vi "Get Control Information.vi"(8 "error in (no error)":errorcluster, 11 "Boolean in":refnum<class "Boolean.lvclass">) -> (0 "error out":errorcluster, 2 "Control Information":string[][](array[string]), 3 "Boolean out":refnum<class "Boolean.lvclass">)   [LabVIEW 2017, in "Localization.lvlib" / "Boolean.lvclass"]
doc: "VI for override that is supposed to do go throgh the process for each control type and pull out the information that is necessary for each control.\n\nChoose Movement Consulting, LLC"
uses:
  Boolean.lvclass
  C:/Apps/CMC/OpenSource/Localization/Control Info/Control Info.lvclass
  Localization.lvlib
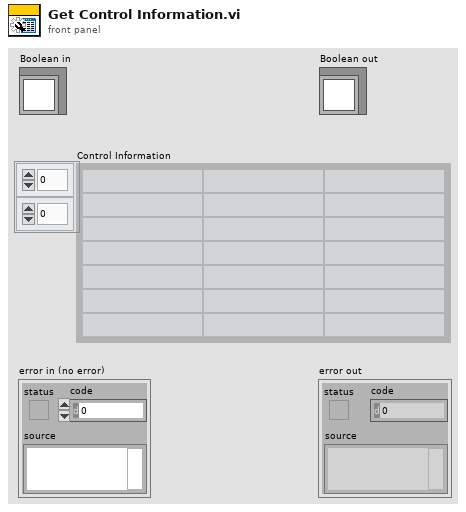
[diagram p1: front panel]
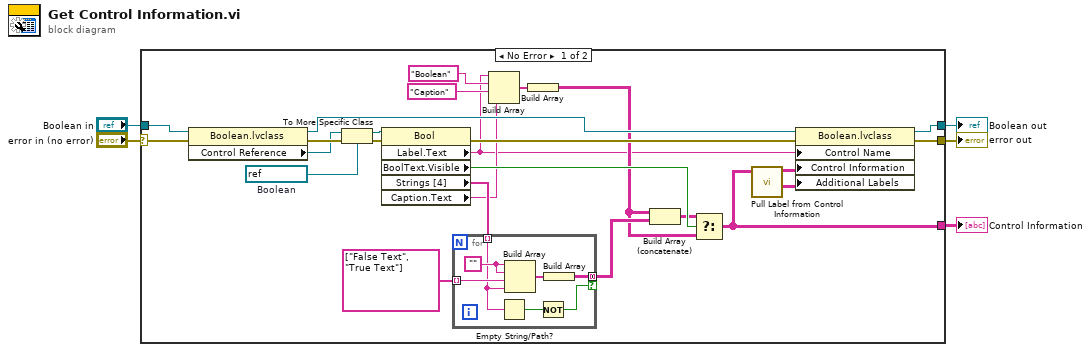
[diagram p0: block diagram]
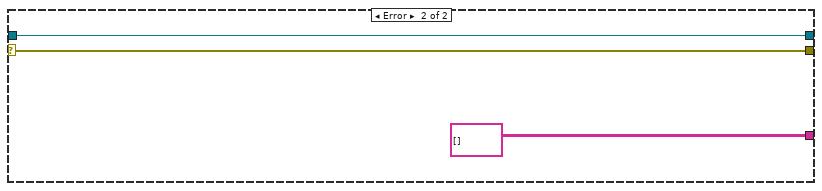
[diagram p2: hidden frame]
diagram:
  n1 = case shown="No Error" "error in (no error)" {
    selector: "error in (no error)" -> [w25 w40]
    tunnel: [w21 w40] -> w1
    tunnel: "Boolean in" -> [w24 w39]
    tunnel: [w9 string[][] []] -> w2
    tunnel: [w19 w39] -> w3
    frame No Error {
      w30 = refnum<vi> refnum  # Boolean
      n2 = property class="Boolean.lvclass"(reference=w24, error in=w25) -> (reference out=w20:refnum<class "Boolean.lvclass">, error out=w26:errorcluster, "Control Reference"=w23:refnum<vi>)
      n3 = To More Specific Class(target class=w30, reference=w23, error in=w26) -> (specific class reference=w29:refnum<vi>, error out=w27:errorcluster)
      n4 = property class="Bool"(reference=w29, error in=w27) -> (error out=w22:errorcluster, "Label.Text"=w6:string, "BoolText.Visible"=w18:bool, "Strings [4]"=w17:string[], "Caption.Text"=w10:string)  [unwired: 1 out]
      n5 = for {
        tunnel: w17 -> [w31] mode=indexing
        tunnel: string[] ["False Text", "True Text"] -> [w33] mode=indexing
        tunnel: [w36] -> w15 mode=concatenating if=w34
        w32 = ""
        n6 = Empty String/Path?(string/path=w31) -> (empty?=w35:bool)
        n7 = Build Array(w32, w32, w33, w31) -> (w37:string[])
        n8 = Not(x=w35) -> (.not. x?=w34:bool)
        n9 = Build Array(w37) -> (w36:string[][])
      }
      n10 = Build Array(w6, "Boolean", "Caption", w10) -> (w28:string[])
      n11 = Build Array(w28) -> (w14:string[][])
      n12 = Build Array (concatenate)(w14, w15) -> (w13:string[][])
      n13 = Select(t=w13, s=w18, f=w14) -> (s? t:f=w9:string[][])
      n14 = call "Pull Label from Control Information.vi"("Control Caption Table"=w9) -> ("Additional Labels"=w7:string[][], "Control Information"=w8:string[][])  [unwired: 9 in]
      n15 = property class="Boolean.lvclass"(reference=w20, error in=w22, "Control Name"=w6, "Control Information"=w8, "Additional Labels"=w7) -> (reference out=w19:refnum<class "Boolean.lvclass">, error out=w21:errorcluster)
    }
    frame Error {
    }
  }
  "error out" <- w1
  "Boolean out" <- w3
  "Control Information" <- w2
